vi "BasicTest.vi"() -> ()   [LabVIEW 2022 SP3]
uses:
  <vilib>/numeric/Random Number (Range) I64.vi
  <vilib>/numeric/sub_Random U32.vi
panel:
  out "Array":string[][](array[string])
  out "Progress":i32(slide) scale=0.0..100.0
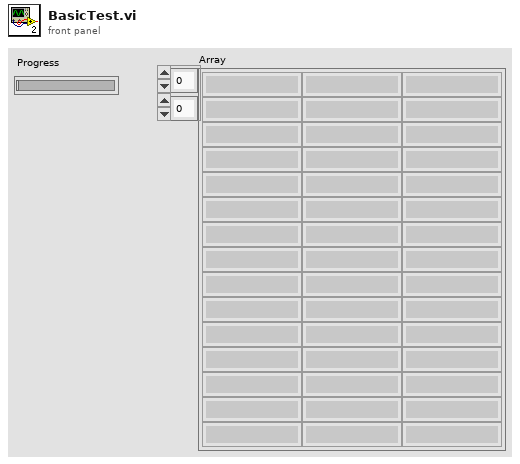
[diagram p1: front panel]
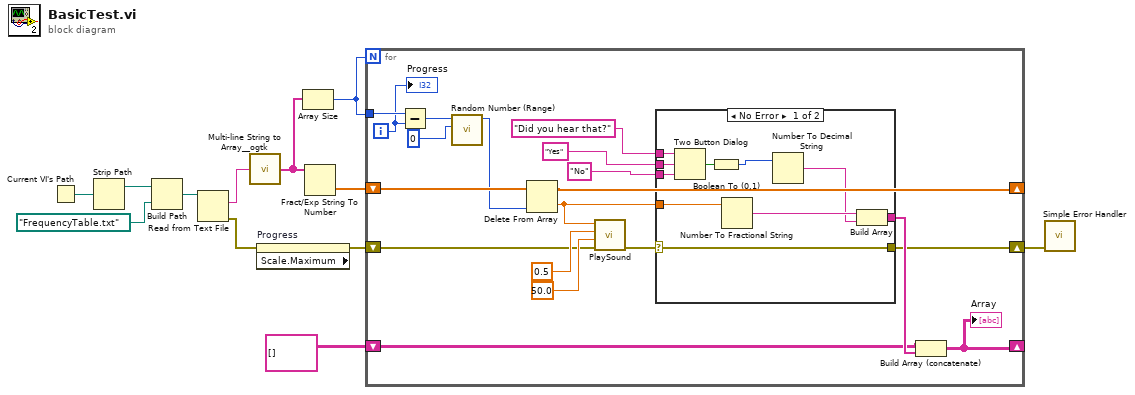
[diagram p0: block diagram]
diagram:
  n1 = Current VI's Path() -> (path=w4:path)
  n2 = Strip Path(path=w4) -> (stripped path=w3:path)  [unwired: 1 out]
  n3 = Build Path(base path=w3, name or relative path=path "FrequencyTable.txt") -> (appended path=w2:path)
  n4 = Read from Text File(file (use dialog)=w2) -> (text=w12:string, error out=w8:errorcluster)  [unwired: 3 in, 2 out]
  n5 = call <userlib>:"Multi-line String to Array__ogtk.vi"("string"=w12) -> ("lines"=w10:string[])
  n6 = property on="Progress" class="Slide (strict)" props=["Scale", "Maximum"](error in=w8) -> (error out=w7:errorcluster)  [unwired: 1 in, 2 out]
  n7 = Array Size(array=w10) -> (size(s)=w9:i32)
  n8 = Fract/Exp String To Number(string=w10) -> (number=w11:dbl[])  [unwired: 3 in, 1 out]
  n9 = for {
    N: w9 -> [_]
    shift-right: [w20] -> _
    shift-left: w11 -> [w28]
    tunnel: w9 -> [w31]
    shift-right: [w13] -> w5
    shift-left: w7 -> [w24]
    shift-right: [w15] -> _
    shift-left: string[][] [] -> [w16]
    i -> [w18]
    n10 = Subtract(x=w31, y=w18) -> (x-y=w30:i32)
    n11 = call-poly <vilib>:"Random Number (Range).vi"("lower bound (-100)"=i64 0, "upper bound (100)"=w30) -> ("number"=w27:i64)  [unwired: 9 in]
    n12 = Delete From Array(array=w28, index=w27) -> (deleted portion=w19:dbl, array with subset deleted=w20:dbl[])  [unwired: 1 in]
    n13 = call "PlaySound.vi"("error in (no error)"=w24, "Volume"=50.0, "Duration (s)"=0.5, "Frequency"=w19) -> ("error out"=w14:errorcluster)  [unwired: 7 in]
    n14 = case shown="No Error" w14 {
      selector: w14 -> [w32 w42]
      tunnel: "Did you hear that?" ("message") -> [w41 _]
      tunnel: "Yes" ("T button name (\"OK\")") -> [w40 _]
      tunnel: "No" ("F button name (\"Cancel\")") -> [w39 _]
      tunnel: w19 -> [w38 _]
      tunnel: [w35 _] -> w17
      tunnel: [w32 w42] -> w13
      frame No Error {
        n15 = Two Button Dialog(message=w41, 1:w39, 2:w40) -> (T button?=w34:bool)
        n16 = Boolean To (0,1)(Boolean=w34) -> (0, 1=w33:i16)
        n17 = Number To Fractional String(number=w38) -> (F-format string=w37:string)  [unwired: 3 in]
        n18 = Number To Decimal String(number=w33) -> (decimal integer string=w36:string)  [unwired: 1 in]
        n19 = Build Array(w37, w36) -> (w35:string[])
      }
      frame Error {
      }
    }
    n20 = Build Array (concatenate)(w16, w17) -> (w15:string[][])
    "Array" <- w15
    "Progress" <- w18
  }
  n21 = call <vilib>:"Simple Error Handler.vi"("error in (no error)"=w5) -> ()  [unwired: 4 in, 5 out]
